vi "GV-MouseDown.vi"(8 "error in (no error)":errorcluster, 9 "Coords":T1, 10 "Button":u16, 11 "Gviewer in":refnum<class "Gviewer.lvclass">) -> (0 "error out":errorcluster, 3 "Gviewer out":refnum<class "Gviewer.lvclass">)   [LabVIEW 2020, in "Sgraph_lib_V1.lvlib" / "Gviewer.lvclass"]
doc: "Andre Koelewijn, 24 jan 2021\n\nAction when in the Gviewer graph the mouse button is pressed."
uses:
  Gviewer.lvclass
  <vilib>/Utility/miscctls.llb/LVPoint32TypeDef.ctl
  Gviewer.lvclass/Gviewer.ctl
  controls/Typedef_Live.ctl
  Common/controls/ToolTypeEnum.ctl
  <vilib>/Utility/cursorutil.llb/Set Cursor (Icon Pict).vi
  Builds/Sgraph_lib_V1.lvlib
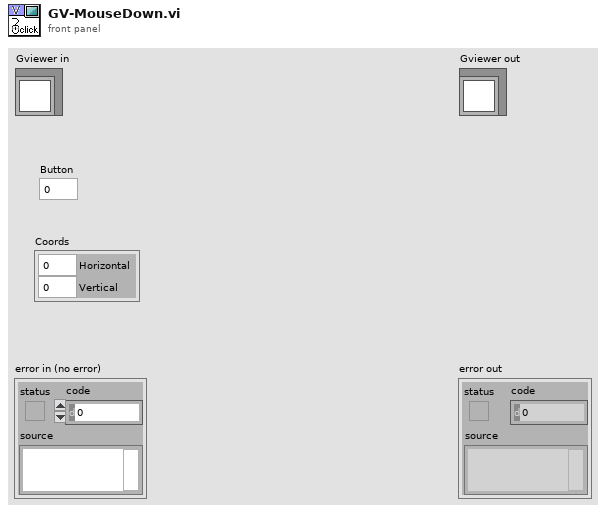
[diagram p1: front panel]
types:
  T1 = typedef "LVPoint32TypeDef.ctl" = cluster{"Horizontal":i32, "Vertical":i32}
  T2 = typedef "Sgraph_lib_V1.lvlib/Gviewer.lvclass/Typedef_Live.ctl" = enum16{"Live View", "Freeze"}
  T3 = typedef "Sgraph_lib_V1.lvlib/ToolTypeEnum.ctl" = enum16{"00_Esc button", "01_Undo", "02_HelpButton", "03_CursorViewButton", "04_AutoScale_Fit", "05_AutoScale_Stacked", "06_ZoomWindowStart", "07_ZoomTimeStart", "08_ZoomAmplitudeStart", "09", "10", "11", "12", "13", "14", "15", "16", "17", "18", "19", "20_VerticalScroll", "21_VerticalMove", "22_TimeScroll", "23_TimeMove", "24", "25", "26_ZoomWindowSize", "27_ZoomTimeWindowSize", "28_ZoomAmplitudeWindowSize", "29", "30_LegendMovePoint", "31_LegendMoveDrag", "32", "33", "34", "35", "36", "37", "38", "39", "40_AddYscalePoint", "41_AddYscalePlace", "42_AddYscaleMovePoint", "43_AddYscaleMoveDrag", "44_AddYscaleDeletePoint"}
  T4 = typedef "Sgraph_lib_V1.lvlib/Gviewer.lvclass/Typedef_SelProperties.ctl" = cluster{"Color":u32, "LineType":T5, "max":dbl, "min":dbl}
  T5 = typedef "Sgraph_lib_V1.lvlib/Gviewer.lvclass/Typedef_LineType.ctl" = enum16{"num_bare", "num_MinMax_Area", "num_MinMax_Lines", "num_MinMax_Forfor", "num_Max_Area", "num_Max_Line", "num_Max_Forfor", "num_Min_Area", "num_Min_Line", "num_Min_Fosfor", "Boolean_Line_01", "Boolean_Area_01", "Boolean_Fosfor_01", "Boolean_Line_TF", "Boolean_Area_TF", "Boolean_Fosfor_TF", "Boolean_OnOff_Line", "Boolean_OnOff_Area", "Boolean_OnOff_Fosfor", "Boolean_spare", "StringEvent_Line", "StringEvent_TimeLine"}
  T6 = typedef "Sgraph_lib_V1.lvlib/Gviewer.lvclass/YgraphDef.ctl" = cluster{"Plot":i32, "X(%)":dbl}
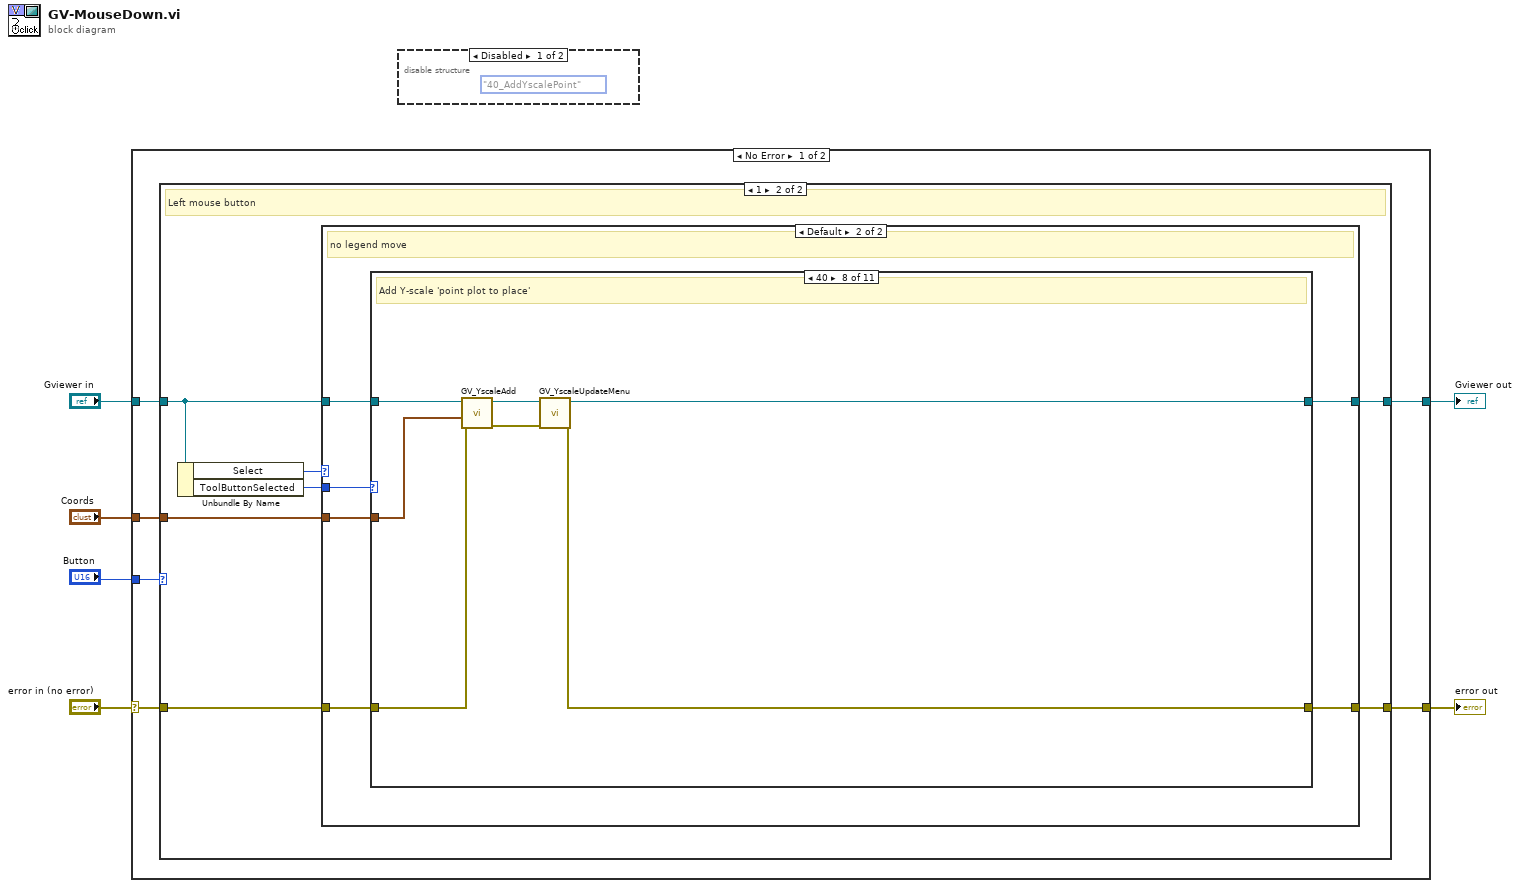
[diagram p0: block diagram]
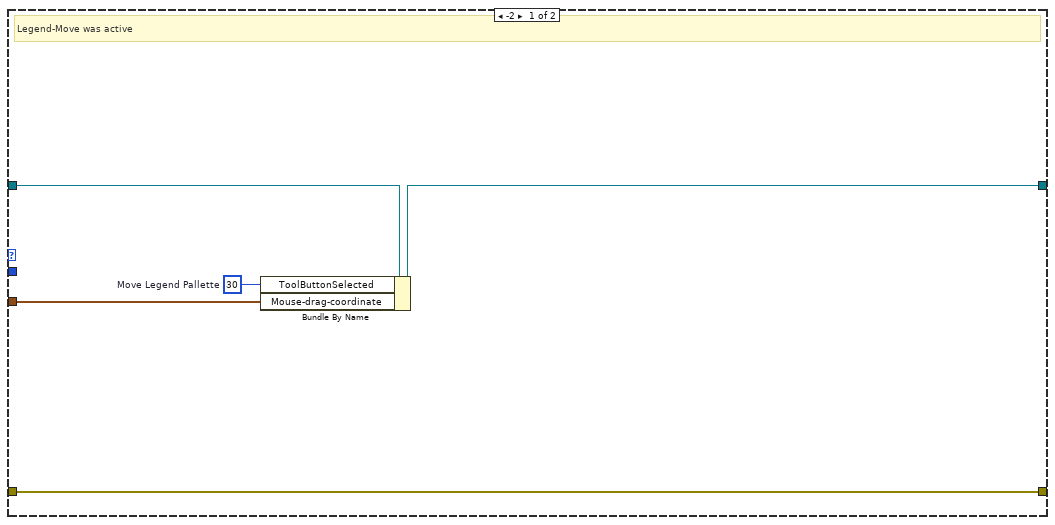
[diagram p4: hidden frame]
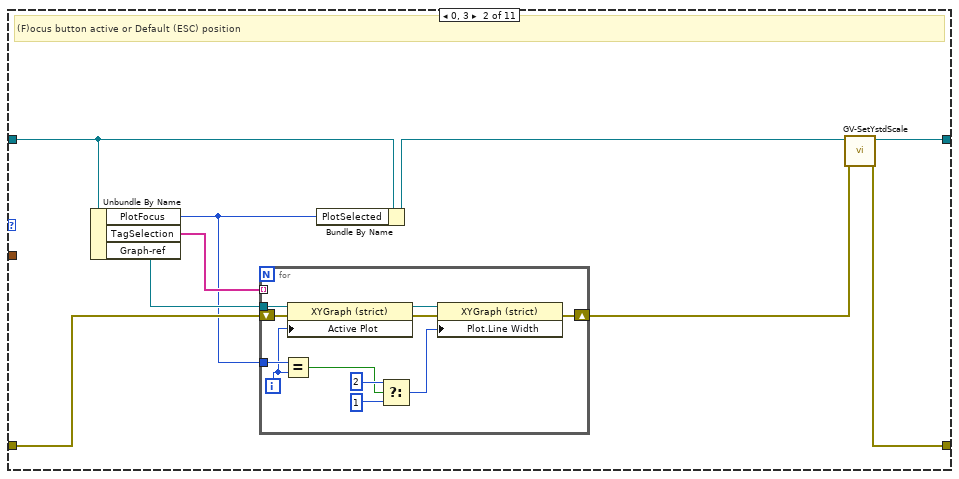
[diagram p6: hidden frame]
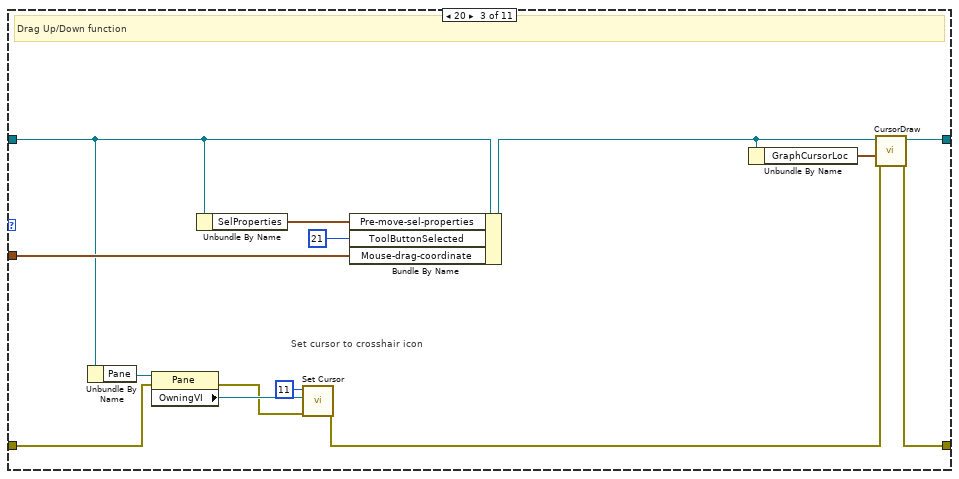
[diagram p7: hidden frame]
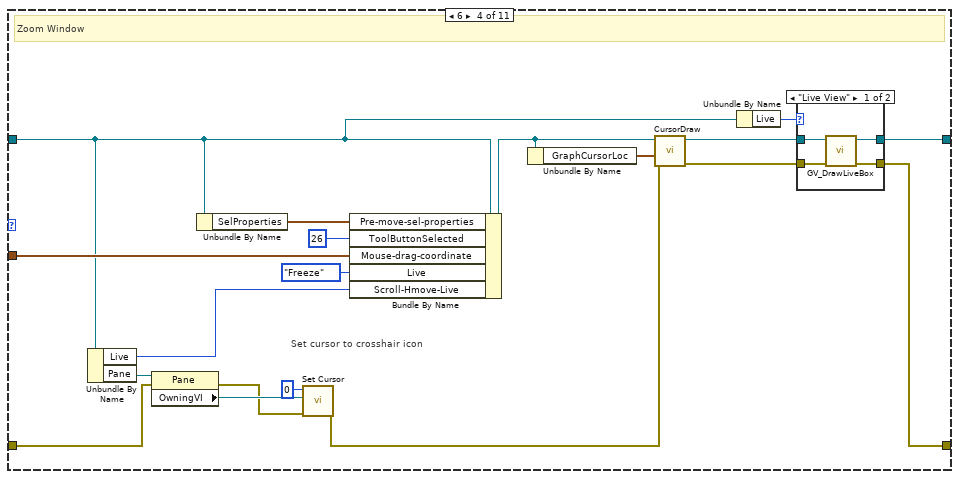
[diagram p8: hidden frame]
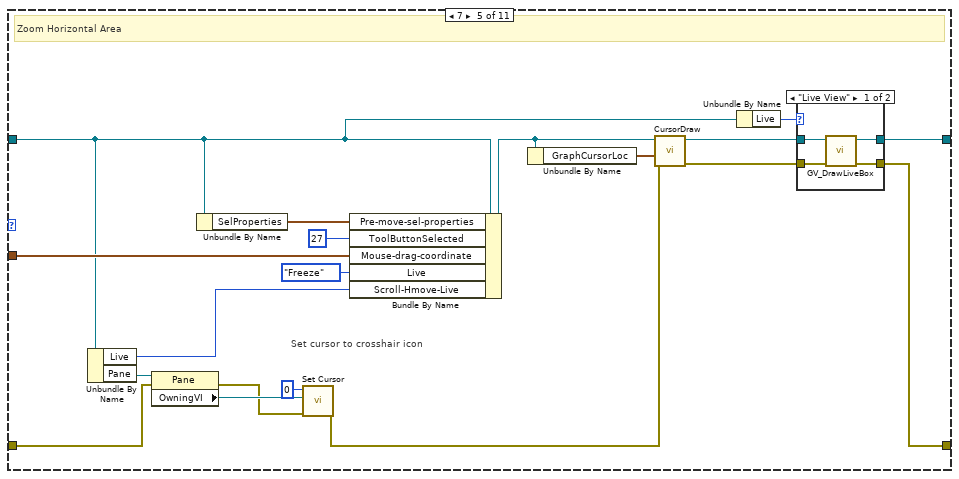
[diagram p10: hidden frame]
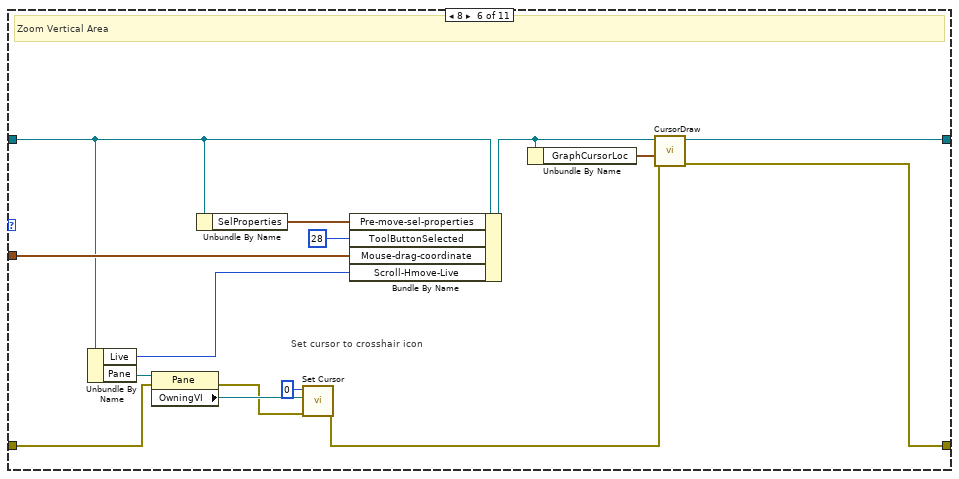
[diagram p12: hidden frame]
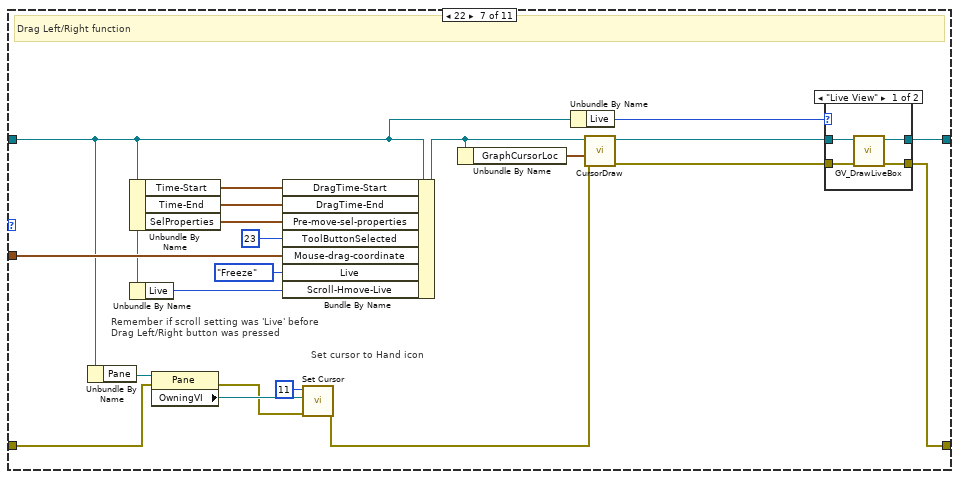
[diagram p13: hidden frame]
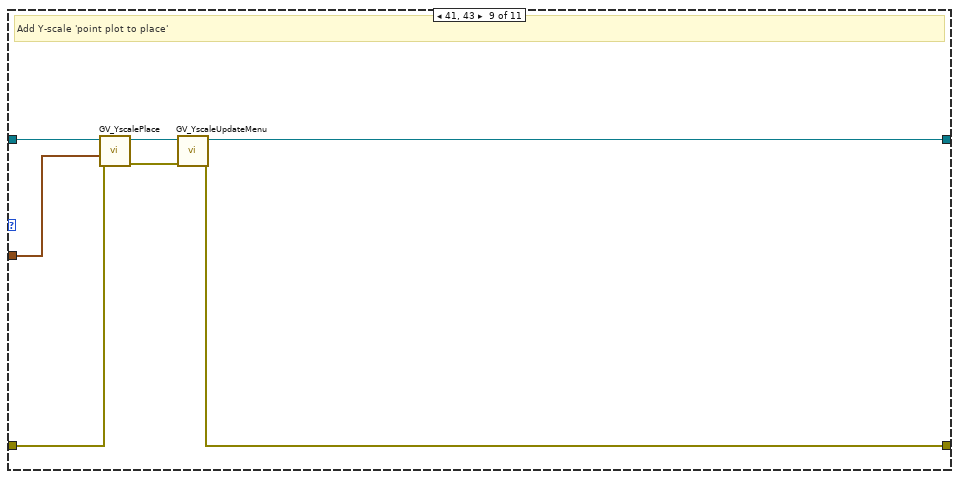
[diagram p15: hidden frame]
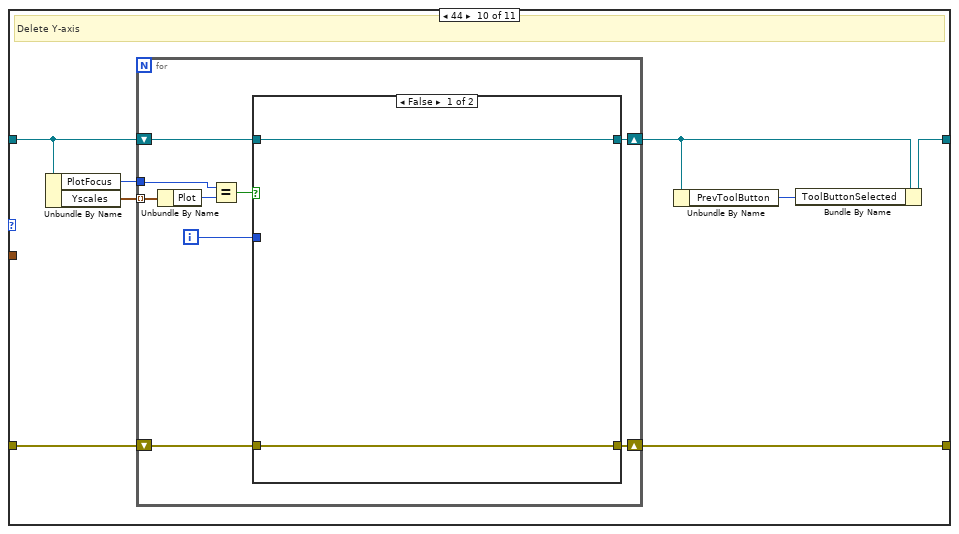
[diagram p16: hidden frame]
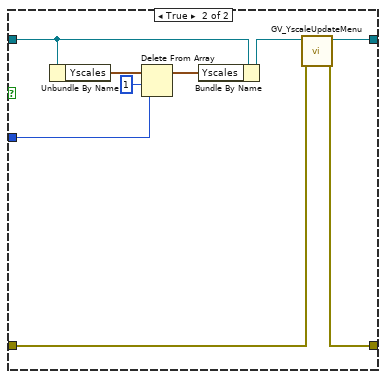
[diagram p17: hidden frame]
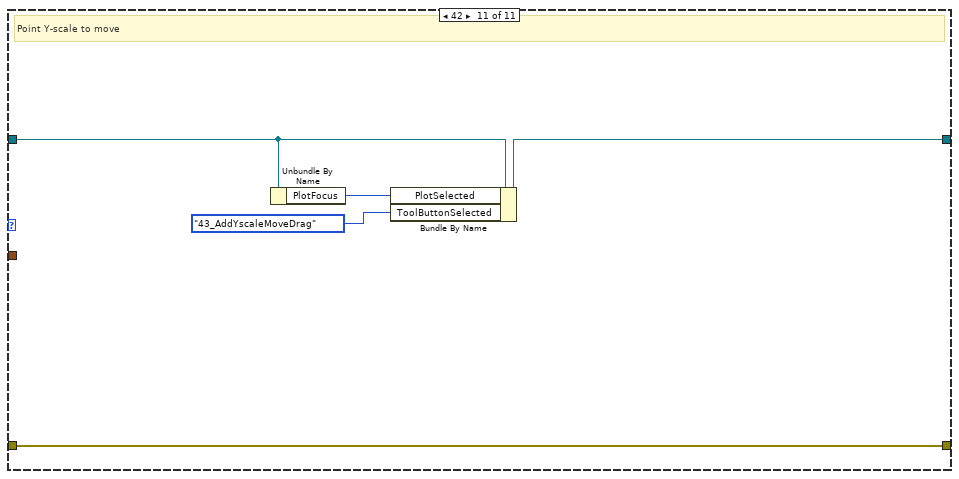
[diagram p18: hidden frame]
diagram:
  n1 = case shown="No Error" "error in (no error)" {
    selector: "error in (no error)" -> [w9 w209]
    tunnel: [w8 w209] -> w5
    tunnel: [w10 w208] -> w3
    tunnel: "Gviewer in" -> [w11 w208]
    tunnel: "Button" -> [w12 _]
    tunnel: "Coords" -> [w7 _]
    frame No Error {
      n2 = case shown="1" w12 {
        tunnel: w11 -> [w14 w20]
        tunnel: [w14 w17] -> w10
        tunnel: w9 -> [w13 w19]
        tunnel: [w13 w18] -> w8
        tunnel: w7 -> [_ w16]
        frame Default {
          # "Other mouse buttons"
        }
        frame 1 {
          # "Left mouse button"
          n3 = Unbundle By Name(w20) -> ("Select"=w15:i32, "ToolButtonSelected"=w21:i32)
          n4 = case shown="Default" w15 {
            tunnel: w21 -> [_ w32]
            tunnel: w20 -> [w24 w31]
            tunnel: w19 -> [w26 w30]
            tunnel: [w26 w29] -> w18
            tunnel: [w25 w28] -> w17
            tunnel: w16 -> [w22 w27]
            frame -2 {
              w23 = 30  # Move Legend Pallette
              # "Legend-Move was active"
              n5 = Bundle By Name(cluster=w24, "ToolButtonSelected"=w23, "Mouse-drag-coordinate"=w22) -> (w25:refnum<class "Gviewer.lvclass">)
            }
            frame Default {
              # "no legend move"
              n6 = case shown="40" w32 {
                tunnel: w31 -> [w34 w42 w61 w71 w96 w122 w137 w167 w174 w182 w204]
                tunnel: w30 -> [w33 w41 w63 w82 w107 w128 w149 w166 w173 w176 w207]
                tunnel: [w33 w38 w55 w75 w100 w119 w139 w163 w170 w175 w207] -> w29
                tunnel: [w34 w39 w57 w77 w102 w120 w141 w161 w168 w177 w205] -> w28
                tunnel: w27 -> [_ _ w62 w81 w106 w127 w148 w165 w172 _ _]
                frame Default {
                  # "other"
                }
                frame 0, 3 {
                  # "(F)ocus button active or Default (ESC) position"
                  n7 = Unbundle By Name(w42) -> ("PlotFocus"=w35:i32, "TagSelection"=w43:string[], "Graph-ref"=w37:refnum<vi>)
                  n8 = for {
                    tunnel: w43 -> [_] mode=indexing
                    tunnel: w35 -> [w46]
                    tunnel: w37 -> [w54]
                    shift-right: [w48] -> w36
                    shift-left: w41 -> [w50]
                    i -> [w45]
                    n9 = Equal?(x=w46, y=w45) -> (x = y?=w47:bool)
                    n10 = property class="XYGraph (strict)"(reference=w54, error in=w50, "Active Plot"=w45) -> (reference out=w53:refnum<vi>, error out=w49:errorcluster)
                    n11 = Select(t=u8 2 ("Plot.Line Width"), s=w47, f=u8 1 ("Plot.Line Width")) -> (s? t:f=w51:u8)
                    n12 = property class="XYGraph (strict)"(reference=w53, error in=w49, "Plot.Line Width"=w51) -> (error out=w48:errorcluster)  [unwired: 1 out]
                  }
                  n13 = Bundle By Name(cluster=w42, "PlotSelected"=w35) -> (w40:refnum<class "Gviewer.lvclass">)
                  n14 = call "GV-SetYstdScale.vi"("error in (no error)"=w36, "Gviewer in"=w40) -> ("error out"=w38:errorcluster, "Gviewer out"=w39:refnum<class "Gviewer.lvclass">)  [unwired: 8 in]
                }
                frame 20 {
                  # "Set cursor to crosshair icon"
                  # "Drag Up/Down function"
                  n15 = Unbundle By Name(w61) -> ("Pane"=w66:refnum<vi>)
                  n16 = property class="Pane"(reference=w66, error in=w63) -> (error out=w64:errorcluster, "OwningVI"=w65:refnum<vi>)  [unwired: 1 out]
                  n17 = Unbundle By Name(w61) -> ("SelProperties"=w60:T4[])
                  n18 = call-poly <vilib>:"Set Cursor.vi"("error in (no error)"=w64, "VI reference (current VI)"=w65, "icon"=u16 11) -> ("error out"=w56:errorcluster)  [unwired: 7 in, 1 out]
                  n19 = Bundle By Name(cluster=w61, "Pre-move-sel-properties"=w60, "ToolButtonSelected"=21, "Mouse-drag-coordinate"=w62) -> (w58:refnum<class "Gviewer.lvclass">)
                  n20 = Unbundle By Name(w58) -> ("GraphCursorLoc"=w59:T1)
                  n21 = call "CursorDraw.vi"("error in (no error)"=w56, "Coords"=w59, "Gviewer in"=w58) -> ("error out"=w55:errorcluster, "Gviewer out"=w57:refnum<class "Gviewer.lvclass">)  [unwired: 7 in]
                }
                frame 6 {
                  # "Set cursor to crosshair icon"
                  # "Zoom Window"
                  n22 = Unbundle By Name(w71) -> ("Live"=w70:T2, "Pane"=w85:refnum<vi>)
                  n23 = property class="Pane"(reference=w85, error in=w82) -> (error out=w83:errorcluster, "OwningVI"=w84:refnum<vi>)  [unwired: 1 out]
                  n24 = Unbundle By Name(w71) -> ("SelProperties"=w80:T4[])
                  n25 = call-poly <vilib>:"Set Cursor.vi"("error in (no error)"=w83, "VI reference (current VI)"=w84, "icon"=u16 0) -> ("error out"=w78:errorcluster)  [unwired: 7 in, 1 out]
                  n26 = Bundle By Name(cluster=w71, "Pre-move-sel-properties"=w80, "ToolButtonSelected"=26, "Mouse-drag-coordinate"=w81, "Live"=Typedef_Live."Freeze", "Scroll-Hmove-Live"=w70) -> (w74:refnum<class "Gviewer.lvclass">)
                  n27 = Unbundle By Name(w74) -> ("GraphCursorLoc"=w79:T1)
                  n28 = call "CursorDraw.vi"("error in (no error)"=w78, "Coords"=w79, "Gviewer in"=w74) -> ("error out"=w76:errorcluster, "Gviewer out"=w72:refnum<class "Gviewer.lvclass">)  [unwired: 7 in]
                  n29 = Unbundle By Name(w71) -> ("Live"=w73:T2)
                  n30 = case shown="\"Live View\"" w73 {
                    tunnel: w72 -> [w91 w93]
                    tunnel: [w90 w93] -> w77
                    tunnel: w76 -> [w89 w92]
                    tunnel: [w88 w92] -> w75
                    frame "Live View" {
                      n31 = call "GV_DrawLiveBox.vi"("error in (no error)"=w89, "Gviewer in"=w91) -> ("error out"=w88:errorcluster, "Gviewer out"=w90:refnum<class "Gviewer.lvclass">)  [unwired: 8 in]
                    }
                    frame "Freeze" {
                    }
                  }
                }
                frame 7 {
                  # "Set cursor to crosshair icon"
                  # "Zoom Horizontal Area"
                  n32 = Unbundle By Name(w96) -> ("Live"=w95:T2, "Pane"=w110:refnum<vi>)
                  n33 = property class="Pane"(reference=w110, error in=w107) -> (error out=w108:errorcluster, "OwningVI"=w109:refnum<vi>)  [unwired: 1 out]
                  n34 = Unbundle By Name(w96) -> ("SelProperties"=w105:T4[])
                  n35 = call-poly <vilib>:"Set Cursor.vi"("error in (no error)"=w108, "VI reference (current VI)"=w109, "icon"=u16 0) -> ("error out"=w103:errorcluster)  [unwired: 7 in, 1 out]
                  n36 = Bundle By Name(cluster=w96, "Pre-move-sel-properties"=w105, "ToolButtonSelected"=27, "Mouse-drag-coordinate"=w106, "Live"=Typedef_Live."Freeze", "Scroll-Hmove-Live"=w95) -> (w99:refnum<class "Gviewer.lvclass">)
                  n37 = Unbundle By Name(w99) -> ("GraphCursorLoc"=w104:T1)
                  n38 = call "CursorDraw.vi"("error in (no error)"=w103, "Coords"=w104, "Gviewer in"=w99) -> ("error out"=w101:errorcluster, "Gviewer out"=w97:refnum<class "Gviewer.lvclass">)  [unwired: 7 in]
                  n39 = Unbundle By Name(w96) -> ("Live"=w98:T2)
                  n40 = case shown="\"Live View\"" w98 {
                    tunnel: w97 -> [w116 w118]
                    tunnel: [w115 w118] -> w102
                    tunnel: w101 -> [w114 w117]
                    tunnel: [w113 w117] -> w100
                    frame "Live View" {
                      n41 = call "GV_DrawLiveBox.vi"("error in (no error)"=w114, "Gviewer in"=w116) -> ("error out"=w113:errorcluster, "Gviewer out"=w115:refnum<class "Gviewer.lvclass">)  [unwired: 8 in]
                    }
                    frame "Freeze" {
                    }
                  }
                }
                frame 8 {
                  # "Set cursor to crosshair icon"
                  # "Zoom Vertical Area"
                  n42 = Unbundle By Name(w122) -> ("Live"=w121:T2, "Pane"=w131:refnum<vi>)
                  n43 = property class="Pane"(reference=w131, error in=w128) -> (error out=w129:errorcluster, "OwningVI"=w130:refnum<vi>)  [unwired: 1 out]
                  n44 = Unbundle By Name(w122) -> ("SelProperties"=w126:T4[])
                  n45 = call-poly <vilib>:"Set Cursor.vi"("error in (no error)"=w129, "VI reference (current VI)"=w130, "icon"=u16 0) -> ("error out"=w124:errorcluster)  [unwired: 7 in, 1 out]
                  n46 = Bundle By Name(cluster=w122, "Pre-move-sel-properties"=w126, "ToolButtonSelected"=28, "Mouse-drag-coordinate"=w127, "Scroll-Hmove-Live"=w121) -> (w123:refnum<class "Gviewer.lvclass">)
                  n47 = Unbundle By Name(w123) -> ("GraphCursorLoc"=w125:T1)
                  n48 = call "CursorDraw.vi"("error in (no error)"=w124, "Coords"=w125, "Gviewer in"=w123) -> ("error out"=w119:errorcluster, "Gviewer out"=w120:refnum<class "Gviewer.lvclass">)  [unwired: 7 in]
                }
                frame 22 {
                  # "Remember if scroll setting was 'Live' before\nDrag Left/Right button was pressed"
                  # "Set cursor to Hand icon"
                  # "Drag Left/Right function"
                  n49 = Unbundle By Name(w137) -> ("Pane"=w152:refnum<vi>)
                  n50 = Unbundle By Name(w137) -> ("Time-Start"=w135:timestamp, "Time-End"=w134:timestamp, "SelProperties"=w147:T4[])
                  n51 = Unbundle By Name(w137) -> ("Live"=w136:T2)
                  n52 = property class="Pane"(reference=w152, error in=w149) -> (error out=w150:errorcluster, "OwningVI"=w151:refnum<vi>)  [unwired: 1 out]
                  n53 = Bundle By Name(cluster=w137, "DragTime-Start"=w135, "DragTime-End"=w134, "Pre-move-sel-properties"=w147, "ToolButtonSelected"=23, "Mouse-drag-coordinate"=w148, "Live"=Typedef_Live."Freeze", "Scroll-Hmove-Live"=w136) -> (w145:refnum<class "Gviewer.lvclass">)
                  n54 = call-poly <vilib>:"Set Cursor.vi"("error in (no error)"=w150, "VI reference (current VI)"=w151, "icon"=u16 11) -> ("error out"=w144:errorcluster)  [unwired: 7 in, 1 out]
                  n55 = Unbundle By Name(w145) -> ("GraphCursorLoc"=w146:T1)
                  n56 = Unbundle By Name(w137) -> ("Live"=w138:T2)
                  n57 = call "CursorDraw.vi"("error in (no error)"=w144, "Coords"=w146, "Gviewer in"=w145) -> ("error out"=w140:errorcluster, "Gviewer out"=w142:refnum<class "Gviewer.lvclass">)  [unwired: 7 in]
                  n58 = case shown="\"Live View\"" w138 {
                    tunnel: w142 -> [w158 w160]
                    tunnel: [w157 w160] -> w141
                    tunnel: w140 -> [w156 w159]
                    tunnel: [w155 w159] -> w139
                    frame "Live View" {
                      n59 = call "GV_DrawLiveBox.vi"("error in (no error)"=w156, "Gviewer in"=w158) -> ("error out"=w155:errorcluster, "Gviewer out"=w157:refnum<class "Gviewer.lvclass">)  [unwired: 8 in]
                    }
                    frame "Freeze" {
                    }
                  }
                }
                frame 40 {
                  # "Add Y-scale 'point plot to place'"
                  n60 = call "GV_YscaleAdd.vi"("error in (no error)"=w166, "Coords"=w165, "Gviewer in"=w167) -> ("error out"=w164:errorcluster, "Gviewer out"=w162:refnum<class "Gviewer.lvclass">)  [unwired: 7 in]
                  n61 = call "GV_YscaleUpdateMenu.vi"("error in (no error)"=w164, "Gviewer in"=w162) -> ("error out"=w163:errorcluster, "Gviewer out"=w161:refnum<class "Gviewer.lvclass">)  [unwired: 8 in]
                }
                frame 41, 43 {
                  # "Add Y-scale 'point plot to place'"
                  n62 = call "GV_YscalePlace.vi"("error in (no error)"=w173, "Coords"=w172, "Gviewer in"=w174) -> ("error out"=w171:errorcluster, "Gviewer out"=w169:refnum<class "Gviewer.lvclass">)  [unwired: 7 in]
                  n63 = call "GV_YscaleUpdateMenu.vi"("error in (no error)"=w171, "Gviewer in"=w169) -> ("error out"=w170:errorcluster, "Gviewer out"=w168:refnum<class "Gviewer.lvclass">)  [unwired: 8 in]
                }
                frame 44 {
                  # "Delete Y-axis"
                  n64 = Unbundle By Name(w182) -> ("PlotFocus"=w180:i32, "Yscales"=w181:T6[])
                  n65 = for {
                    shift-right: [w187] -> w178
                    shift-left: w182 -> [w188]
                    tunnel: w181 -> [w191] mode=indexing
                    tunnel: w180 -> [w186]
                    shift-right: [w183] -> w175
                    shift-left: w176 -> [w184]
                    i -> [w185]
                    n66 = Unbundle By Name(w191) -> ("Plot"=w190:i32)
                    n67 = Equal?(x=w186, y=w190) -> (x = y?=w189:bool)
                    n68 = case shown="False" w189 {
                      tunnel: w188 -> [w193 w200]
                      tunnel: [w193 w196] -> w187
                      tunnel: w185 -> [_ w198]
                      tunnel: w184 -> [w192 w195]
                      tunnel: [w192 w194] -> w183
                      frame False {
                      }
                      frame True {
                        n69 = Unbundle By Name(w200) -> ("Yscales"=w202:T6[])
                        n70 = Delete From Array(array=w202, length=1, index=w198) -> (array with subset deleted=w199:T6[])  [unwired: 1 out]
                        n71 = Bundle By Name(cluster=w200, "Yscales"=w199) -> (w197:refnum<class "Gviewer.lvclass">)
                        n72 = call "GV_YscaleUpdateMenu.vi"("error in (no error)"=w195, "Gviewer in"=w197) -> ("error out"=w194:errorcluster, "Gviewer out"=w196:refnum<class "Gviewer.lvclass">)  [unwired: 8 in]
                      }
                    }
                  }
                  n73 = Unbundle By Name(w178) -> ("PrevToolButton"=w179:i32)
                  n74 = Bundle By Name(cluster=w178, "ToolButtonSelected"=w179) -> (w177:refnum<class "Gviewer.lvclass">)
                }
                frame 42 {
                  # "Point Y-scale to move"
                  n75 = Unbundle By Name(w204) -> ("PlotFocus"=w206:i32)
                  n76 = Bundle By Name(cluster=w204, "PlotSelected"=w206, "ToolButtonSelected"=ToolTypeEnum."43_AddYscaleMoveDrag" ("Enum")) -> (w205:refnum<class "Gviewer.lvclass">)
                }
              }
            }
          }
        }
      }
    }
    frame Error {
    }
  }
  "error out" <- w5
  "Gviewer out" <- w3
  n77 = disable-structure shown="Disabled" {
    frame Disabled {
      (unwired) ToolTypeEnum."40_AddYscalePoint" ("Enum")
    }
    frame Enabled {
    }
  }
